vi "IntakeDash_WriteTuning.vi"(4 "AlgaeSensorOffDelaySec":dbl, 6 "AlgaeSensorOnDelaySec":dbl, 9 "AlgaeIntakeMtr":dbl, 11 "AlgaeHoldMtr":dbl) -> ()   [LabVIEW 2023]
uses:
  <vilib>/Rock Robotics/Network Tables/NT Write Number.vi
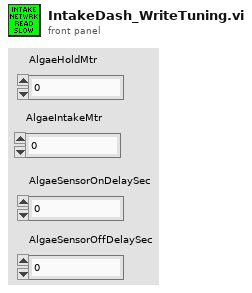
[diagram p1: front panel]
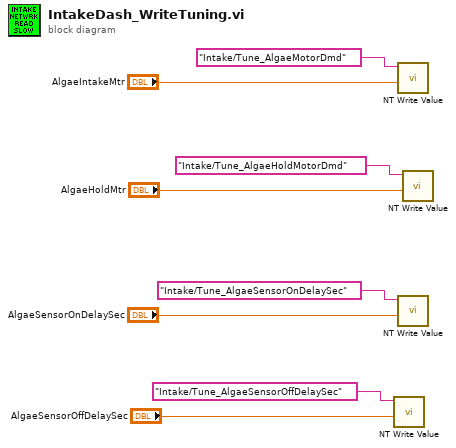
[diagram p0: block diagram]
diagram:
  n1 = call-poly <vilib>:"NT Write Value.vi"("value"="AlgaeSensorOffDelaySec", "name"="Intake/Tune_AlgaeSensorOffDelaySec") -> ()  [unwired: 9 in, 1 out]
  n2 = call-poly <vilib>:"NT Write Value.vi"("value"="AlgaeIntakeMtr", "name"="Intake/Tune_AlgaeMotorDmd") -> ()  [unwired: 9 in, 1 out]
  n3 = call-poly <vilib>:"NT Write Value.vi"("value"="AlgaeSensorOnDelaySec", "name"="Intake/Tune_AlgaeSensorOnDelaySec") -> ()  [unwired: 9 in, 1 out]
  n4 = call-poly <vilib>:"NT Write Value.vi"("value"="AlgaeHoldMtr", "name"="Intake/Tune_AlgaeHoldMotorDmd") -> ()  [unwired: 9 in, 1 out]
